vi "Switch lockin settings.vi"() -> ()   [LabVIEW 2016]
uses:
  <userlib>/LevyLab/Lockin-Multichannel/Typedefs/AO-cluster.ctl
  <userlib>/LevyLab/Lockin-Multichannel/Typedefs/AO_Amp-array.ctl
  <userlib>/LevyLab/Lockin-Multichannel/Typedefs/AO_DC-array.ctl
  <userlib>/LevyLab/Lockin-Multichannel/Typedefs/AO_f-array.ctl
  <userlib>/LevyLab/Lockin-Multichannel/Typedefs/AO_phi-array.ctl
  <userlib>/LevyLab/Lockin-Multichannel/Typedefs/Function-array.ctl
  <userlib>/LevyLab/Lockin-Multichannel/Typedefs/Function-enum.ctl
panel:
  in  "Channel":i32[](array[numeric])
  in  "output cluster 2":T1={"AO amp (V)"=[0.01, 0.0, 0.0, 0.0, 0.0, 0.0, 0.0, 0.0], "AO DC (V)"=[0.0, 0.0, 0.0, 0.0, 0.0, 0.0, 0.0, 0.0], "AO f (Hz)"=[13.1, 13.0, 13.0, 13.0, 13.0, 13.0, 13.0, 13.0], "AO phi (deg)"=[0.0, 0.0, 0.0, 0.0, 0.0, 0.0, 0.0, 0.0], "function"=[enum."Sine Wave", enum."Sine Wave", enum."Sine Wave", enum."Sine Wave", enum."Sine Wave", enum."Sine Wave", enum."Sine Wave", enum."Sine Wave"]} {"AO f (Hz)" min=0.001 max=10000.0; "AO DC (V)" format="%#_6p"; "AO amp (V)" format="%#_6p"}
  out "error out":errorcluster
  out "reference out":refnum<vi>
  in  "Initial settings for Channels: AO":T1={"AO amp (V)"=[0.0, 0.0, 0.0, 0.0, 0.0, 0.0, 0.0, 0.0], "AO DC (V)"=[0.0, 0.0, 0.0, 0.0, 0.0, 0.0, 0.0, 0.0], "AO f (Hz)"=[13.0, 13.0, 13.0, 13.0, 13.0, 13.0, 13.0, 13.0], "AO phi (deg)"=[0.0, 0.0, 0.0, 0.0, 0.0, 0.0, 0.0, 0.0], "function"=[enum."Sine Wave", enum."Sine Wave", enum."Sine Wave", enum."Sine Wave", enum."Sine Wave", enum."Sine Wave", enum."Sine Wave", enum."Sine Wave"]} {"AO f (Hz)" min=0.001 max=10000.0; "AO DC (V)" format="%#_6p"; "AO amp (V)" format="%#_6p"}
  out "output cluster":T1={"AO amp (V)"=[0.01, 0.0, 0.0, 0.0, 0.0, 0.0, 0.0, 0.0], "AO DC (V)"=[0.0, 0.0, 0.0, 0.0, 0.0, 0.0, 0.0, 0.0], "AO f (Hz)"=[13.1, 13.0, 13.0, 13.0, 13.0, 13.0, 13.0, 13.0], "AO phi (deg)"=[0.0, 0.0, 0.0, 0.0, 0.0, 0.0, 0.0, 0.0], "function"=[enum."Sine Wave", enum."Sine Wave", enum."Sine Wave", enum."Sine Wave", enum."Sine Wave", enum."Sine Wave", enum."Sine Wave", enum."Sine Wave"]} {"AO f (Hz)" min=0.001 max=10000.0; "AO DC (V)" format="%#_6p"; "AO amp (V)" format="%#_6p"}
  in  "Recipe row you want to choose":i32
  # "0"
  # "1"
  # "2"
  # "3"
  # "4"
  # "5"
  # "6"
  # "7"
  # "0"
  # "1"
  # "2"
  # "3"
  # "4"
  # "5"
  # "6"
  # "7"
  # "0"
  # "1"
  # "2"
  # "3"
  # "4"
  # "5"
  # "6"
  # "7"
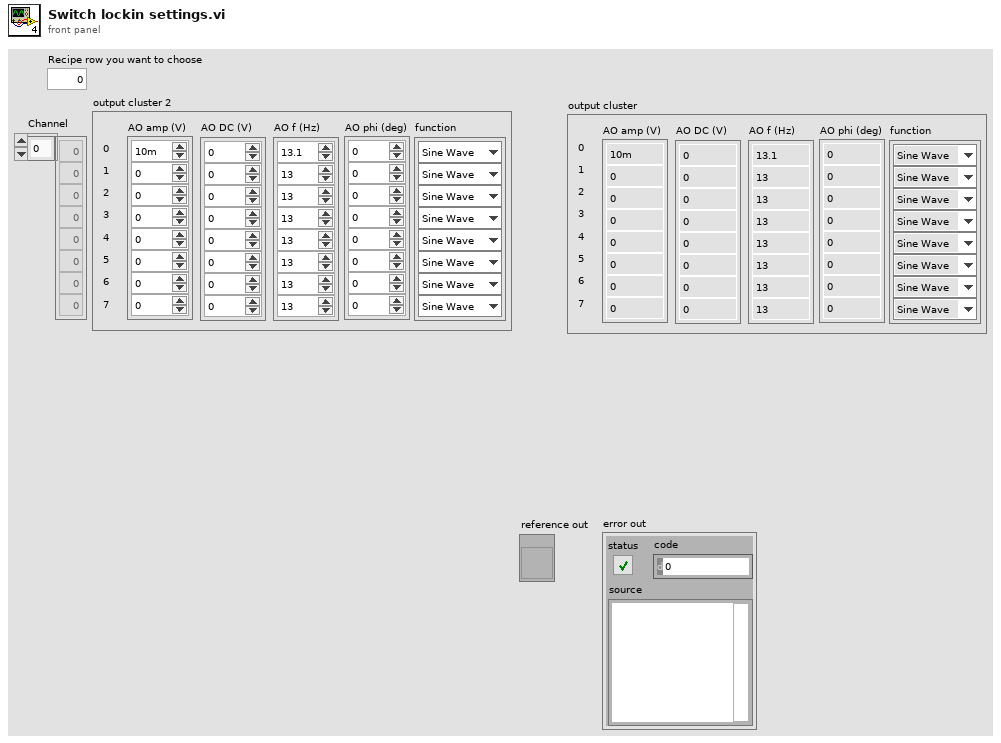
[diagram p1: front panel]
types:
  T1 = typedef "AO-cluster.ctl" = cluster{"AO amp (V)":T2, "AO DC (V)":T3, "AO f (Hz)":T4, "AO phi (deg)":T5, "function":T6}
  T2 = typedef "AO_Amp-array.ctl" = dbl[]
  T3 = typedef "AO_DC-array.ctl" = dbl[]
  T4 = typedef "AO_f-array.ctl" = dbl[]
  T5 = typedef "AO_phi-array.ctl" = dbl[]
  T6 = typedef "Function-array.ctl" = T7[]
  T7 = typedef "Function-enum.ctl" = enum16{"Sine Wave", "Triangle Wave", "Square Wave", "Sawtooth Wave"}
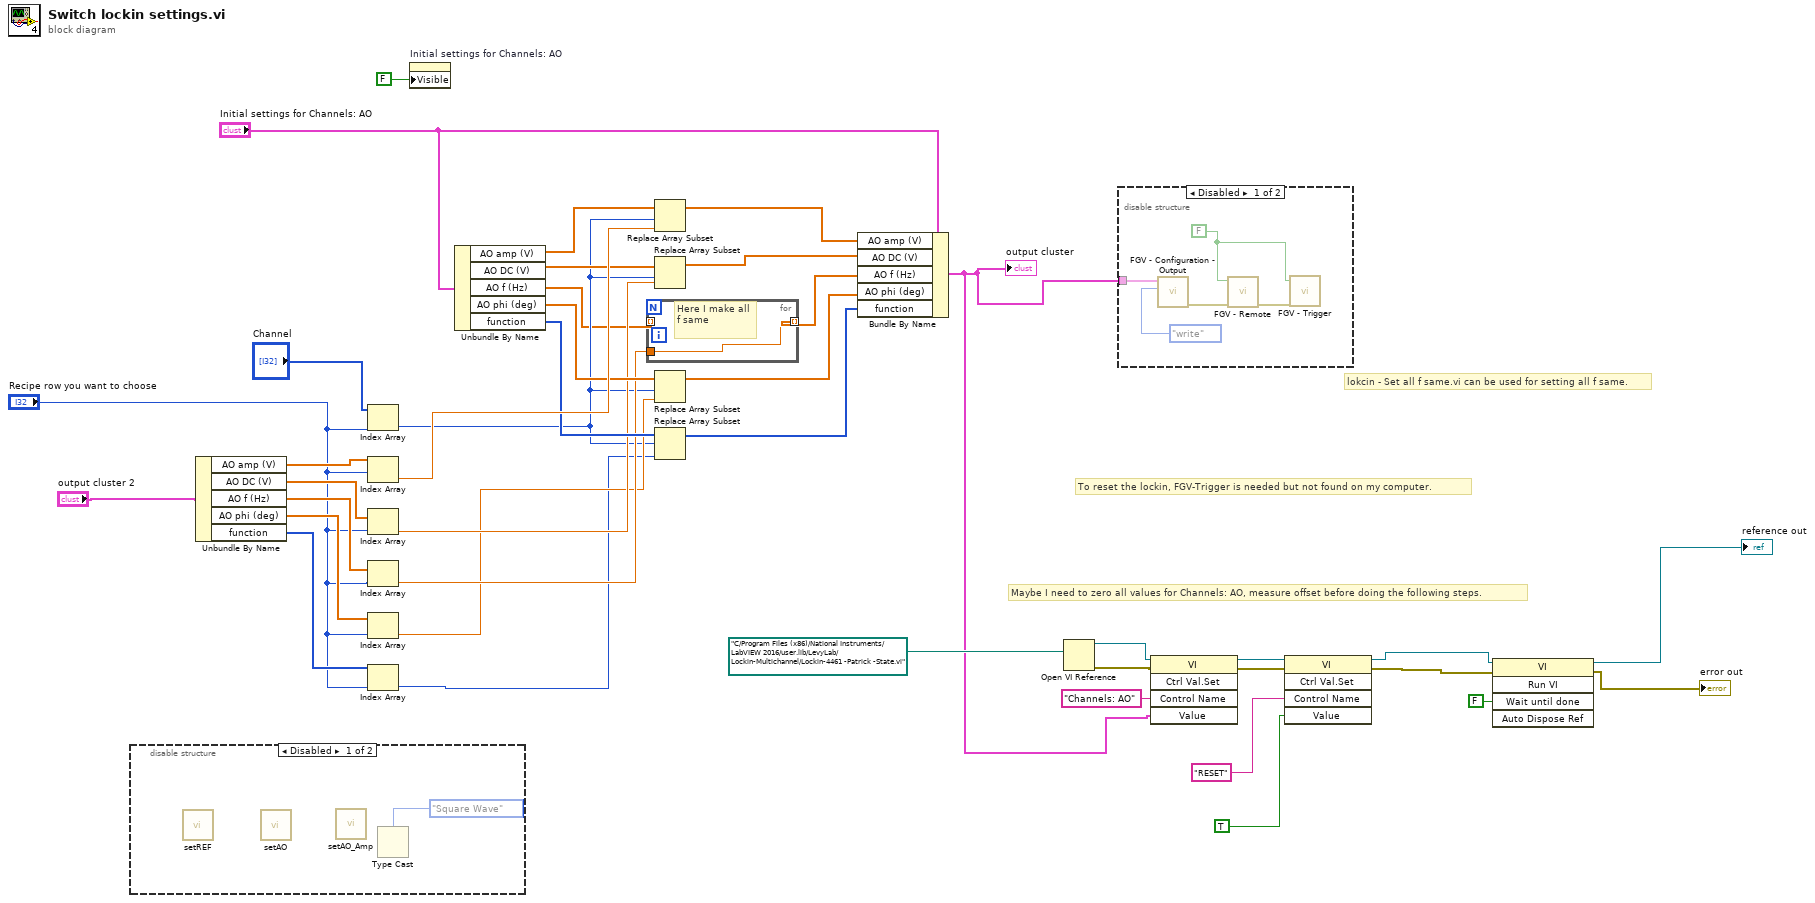
[diagram p0: block diagram]
diagram:
  # "Maybe I need to zero all values for Channels: AO, measure offset before doing the following steps."
  # "lokcin - Set all f same.vi can be used for setting all f same."
  # "To reset the lockin, FGV-Trigger is needed but not found on my computer."
  n1 = disable-structure shown="Disabled" {
    frame Disabled {
      n2 = call <userlib>:"setREF.vi"() -> ()  [unwired: 10 in, 2 out]
      n3 = call <userlib>:"setAO.vi"() -> ()  [unwired: 10 in, 2 out]
      n4 = call <userlib>:"setAO_Amp.vi"() -> ()  [unwired: 10 in, 2 out]
      n5 = Type Cast(type=Function-enum."Square Wave" ("Signal Type")) -> ()  [unwired: 1 in, 1 out]
    }
    frame Enabled {
    }
  }
  n6 = Unbundle By Name("output cluster 2") -> ("AO amp (V)"=w40:T2, "AO DC (V)"=w39:T3, "AO f (Hz)"=w38:T4, "AO phi (deg)"=w37:T5, "function"=w36:T6)
  n7 = Index Array(array="Channel", index="Recipe row you want to choose") -> (element=w27:i32)
  n8 = Index Array(array=w40, index="Recipe row you want to choose") -> (element=w34:dbl)
  n9 = Index Array(array=w39, index="Recipe row you want to choose") -> (element=w30:dbl)
  n10 = Index Array(array=w38, index="Recipe row you want to choose") -> (element=w29:dbl)
  n11 = Index Array(array=w37, index="Recipe row you want to choose") -> (element=w28:dbl)
  n12 = Index Array(array=w36, index="Recipe row you want to choose") -> (element=w3:T7)
  n13 = property on="Initial settings for Channels: AO" class="Clust (strict)"("Visible"=FALSE) -> ()  [unwired: 2 in, 2 out]
  n14 = Unbundle By Name("Initial settings for Channels: AO") -> ("AO amp (V)"=w35:T2, "AO DC (V)"=w33:T3, "AO f (Hz)"=w20:T4, "AO phi (deg)"=w32:T5, "function"=w31:T6)
  n15 = for {
    tunnel: w20 -> [_] mode=indexing
    tunnel: w29 -> [w42]
    tunnel: [w42] -> w19 mode=indexing
    # "Here I make all f same"
  }
  n16 = Replace Array Subset(array=w35, new element=w34, index=w27) -> (w26:T2)
  n17 = Replace Array Subset(array=w33, new element=w30, index=w27) -> (w25:T3)
  n18 = Replace Array Subset(array=w32, new element=w28, index=w27) -> (w24:T5)
  n19 = Replace Array Subset(array=w31, new element=w3, index=w27) -> (w23:T6)
  n20 = Bundle By Name(cluster="Initial settings for Channels: AO", "AO amp (V)"=w26, "AO DC (V)"=w25, "AO f (Hz)"=w19, "AO phi (deg)"=w24, "function"=w23) -> (w7:T1)
  "output cluster" <- w7
  n21 = Open VI Reference(vi path=path "C:/Program Files (x86)/National Instruments/LabVIEW 2016/user.lib/LevyLab/Lockin-Multichannel/Lockin-4461 -Patrick -State.vi") -> (vi reference=w16:refnum<vi>, error out=w15:errorcluster)  [unwired: 5 in]
  n22 = disable-structure shown="Disabled" {
    disable-tunnel: w7 -> [w43 _]
    frame Disabled {
      w44 = FALSE ("Remote Mode")
      n23 = call <userlib>:"FGV - Configuration - Output.vi"("Function"=enum16{"write", "read"}."write", "Channels: AO"=w43) -> ("error out"=w46:errorcluster)  [unwired: 4 in, 1 out]
      n24 = call <userlib>:"FGV - Remote.vi"("error in"=w46, "Remote Mode"=w44) -> ("error out"=w45:errorcluster)  [unwired: 4 in, 1 out]
      n25 = call <userlib>:"FGV - Trigger.vi"("error in"=w45, "Trigger"=w44) -> ()  [unwired: 4 in, 2 out]
    }
    frame Enabled {
    }
  }
  n26 = invoke class="VI" method="Ctrl Val.Set"(reference=w16, error in=w15, "Control Name"="Channels: AO", "Value"=w7) -> (reference out=w13:refnum<vi>, error out=w14:errorcluster)  [unwired: 1 in, 3 out]
  n27 = invoke class="VI" method="Ctrl Val.Set"(reference=w13, error in=w14, "Control Name"="RESET", "Value"=TRUE ("Wait Until Done")) -> (reference out=w10:refnum<vi>, error out=w11:errorcluster)  [unwired: 1 in, 3 out]
  n28 = invoke class="VI" method="Run VI"(reference=w10, error in=w11, "Wait until done"=FALSE ("Wait Until Done")) -> (reference out=→"reference out":refnum<vi>, error out=→"error out":errorcluster)  [unwired: 2 in, 3 out]
